vi "SPCControls.vi"(1 "Set/Get":bool, 2 "Control References (input)":refnum<vi>[](array[refnum])) -> (0 "Control References (output)":refnum<vi>[](array[refnum]))   [LabVIEW 2009]
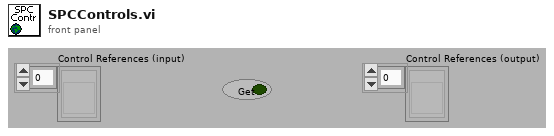
[diagram p1: front panel]
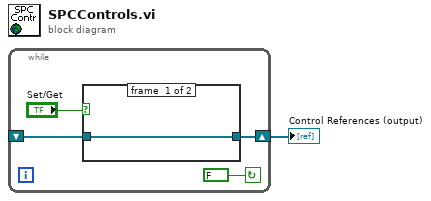
[diagram p0: block diagram]
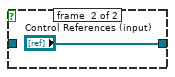
[diagram p2: hidden frame]
diagram:
  n1 = while {
    shift-right: [w4] -> w1
    shift-left: _ -> [w3]
    stop <- FALSE continue-if-true
    n2 = case shown="False" "Set/Get" {
      tunnel: [w6 "Control References (input)"] -> w4
      tunnel: w3 -> [w6 _]
      frame #0 {
      }
      frame #1 {
      }
    }
  }
  "Control References (output)" <- w1
